vi "GET_2D_Data_Binning_(location).vi"(4 "Y":dbl[](array[numeric]), 5 "X":dbl[](array[numeric]), 6 "Bins parameters":T1={"Xmax"=110.0, "Xmin"=-110.0, "Ymax"=110.0, "Ymin"=-110.0, "# bins per axis"=64}) -> (2 "Binned array":u32[][](array[numeric]))   [LabVIEW 2018, in "Tracker.lvlib"]
uses:
  Tracker.lvlib
  Controls/CTL_2D_bins_parameters.ctl
panel:
  out "Y bins (center)":dbl[](array[numeric])
  out "X bins (center)":dbl[](array[numeric])
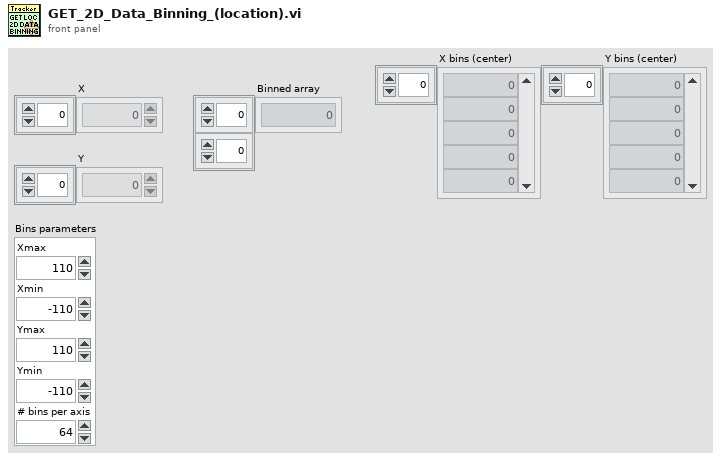
[diagram p1: front panel]
types:
  T1 = typedef "Tracker.lvlib/CTL_2D_bins_parameters.ctl" = cluster{"Xmax":dbl, "Xmin":dbl, "Ymax":dbl, "Ymin":dbl, "# bins per axis":i32}
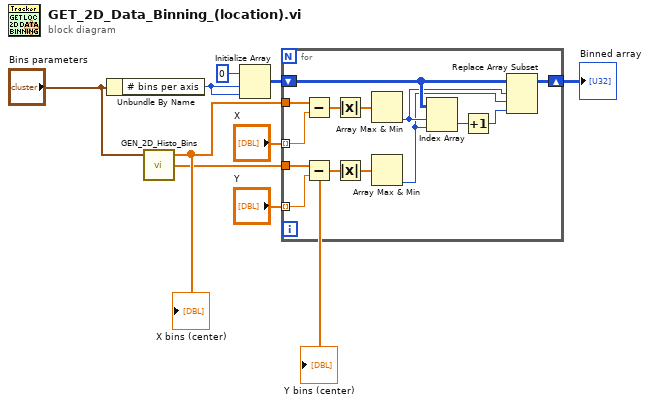
[diagram p0: block diagram]
diagram:
  n1 = Unbundle By Name("Bins parameters") -> ("# bins per axis"=w2:i32)
  n2 = call "GEN_2D_Histo_Bins.vi"("Bins parameters"="Bins parameters") -> ("Y bins (center)"=w8:dbl[], "X bins (center)"=w9:dbl[])  [unwired: 2 in, 1 out]
  "X bins (center)" <- w9
  "Y bins (center)" <- w8
  n3 = Initialize Array(u32 0, w2, w2) -> (w6:u32[][])
  n4 = for {
    tunnel: "X" -> [w22] mode=indexing
    tunnel: "Y" -> [w19] mode=indexing
    tunnel: w9 -> [w23]
    tunnel: w8 -> [w18]
    shift-right: [w15] -> w1
    shift-left: w6 -> [w17]
    n5 = Subtract(x=w23, y=w22) -> (x-y=w21:dbl[])
    n6 = Subtract(x=w18, y=w19) -> (x-y=w20:dbl[])
    n7 = Absolute Value(x=w21) -> (abs(x)=w13:dbl[])
    n8 = Absolute Value(x=w20) -> (abs(x)=w12:dbl[])
    n9 = Array Max & Min(array=w13) -> (min index (indices)=w11:i32)  [unwired: 3 out]
    n10 = Array Max & Min(array=w12) -> (min index (indices)=w10:i32)  [unwired: 3 out]
    n11 = Index Array(array=w17, index (row)=w11, index (col)=w10) -> (element=w16:u32)
    n12 = Increment(x=w16) -> (x+1=w14:u32)
    n13 = Replace Array Subset(array=w17, new element=w14, index (row)=w11, index (col)=w10) -> (w15:u32[][])
  }
  "Binned array" <- w1
